vi "LinkParticles.vi"(4 "Fixed Size":bool=TRUE, 6 "Accept New":bool=TRUE, 10 "New Particle Positions":dbl[][](array[numeric])=[[305.5627746582031, 67.89103698730469], [341.9431457519531, 72.40214538574219], [232.1138153076172, 91.70089721679688], [411.30303955078125, 99.19172668457031], [201.31768798828125, 112.402099609375], [178.73162841796875, 140.29721069335938], [455.8645935058594, 155.0275421142578], [163.60015869140625, 176.1148223876953], [154.8563995361328, 211.54965209960938], [476.7146911621094, 222.72250366210938], [37.367530822753906, 236.38706970214844], [157.02395629882812, 249.5926971435547], [167.57664489746094, 281.2937927246094], [460.26348876953125, 297.98388671875], [184.57943725585938, 313.2145690917969], [442.5791320800781, 331.2660827636719], [206.3518829345703, 345.27783203125], [415.7437438964844, 355.53765869140625], [239.37156677246094, 369.4365539550781], [382.6512451171875, 372.81396484375], [268.6066589355469, 375.957275390625], [345.42205810546875, 383.692626953125], [307.2210388183594, 390.125], [315.5556335449219, 454.518798828125], [261.72613525390625, 461.53814697265625], [399.8280944824219, 466.7994079589844], [450.890869140625, 478.2618103027344]], 11 "Old Particle Positions":dbl[][](array[numeric])=[[305.5627746582031, 67.89103698730469], [341.9431457519531, 72.40214538574219], [232.1138153076172, 91.70089721679688], [411.30303955078125, 99.19172668457031], [201.31768798828125, 112.402099609375], [178.73162841796875, 140.29721069335938], [455.8645935058594, 155.0275421142578], [163.60015869140625, 176.1148223876953], [154.8563995361328, 211.54965209960938], [476.7146911621094, 222.72250366210938], [37.367530822753906, 236.38706970214844], [157.02395629882812, 249.5926971435547], [167.57664489746094, 281.2937927246094], [460.26348876953125, 297.98388671875], [184.57943725585938, 313.2145690917969], [442.5791320800781, 331.2660827636719], [206.3518829345703, 345.27783203125], [415.7437438964844, 355.53765869140625], [239.37156677246094, 369.4365539550781], [382.6512451171875, 372.81396484375], [268.6066589355469, 375.957275390625], [345.42205810546875, 383.692626953125], [307.2210388183594, 390.125], [315.5556335449219, 454.518798828125], [261.72613525390625, 461.53814697265625], [399.8280944824219, 466.7994079589844], [450.890869140625, 478.2618103027344]]) -> (3 "New Particle Positions Out":dbl[][](array[numeric]))   [LabVIEW 2017, in "ImageAcquisitionLibrary.lvlib"]
uses:
  ImageAcquisitionLibrary.lvlib
panel:
  out "Array":i32[](array[numeric])
  out "Distances":dbl[][](array[numeric])
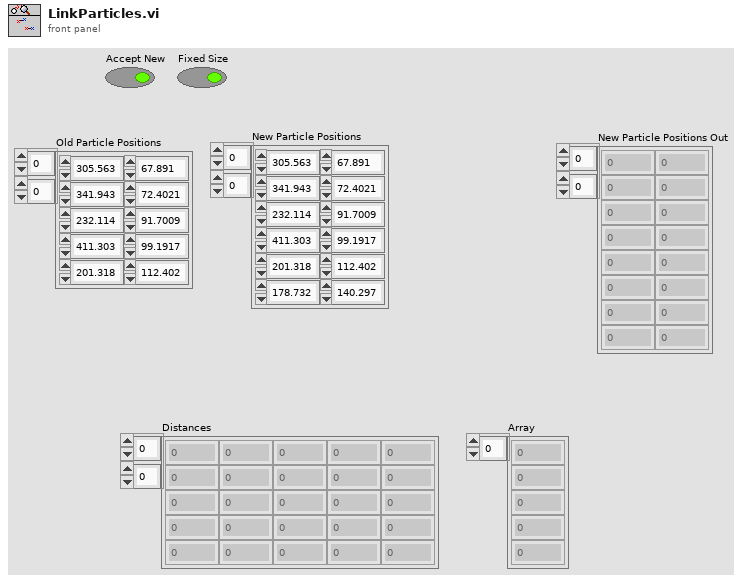
[diagram p1: front panel]
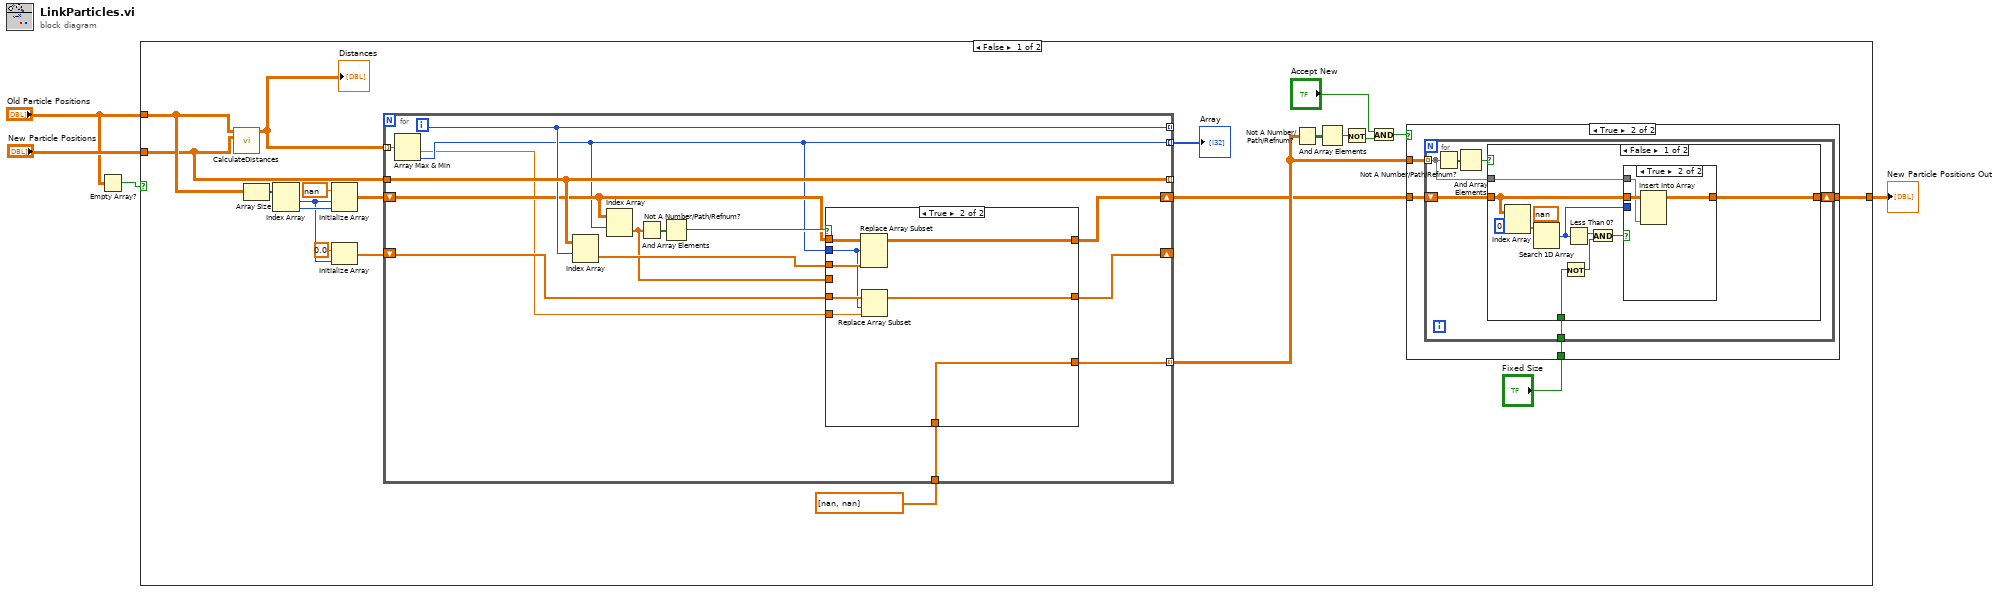
[diagram p0: block diagram]
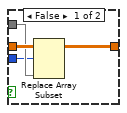
[diagram p3: hidden frame]
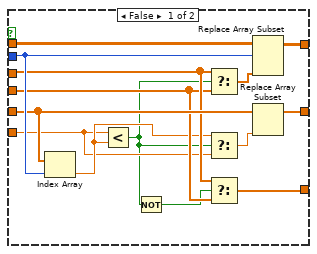
[diagram p5: hidden frame]
diagram:
  n1 = Empty Array?(array="Old Particle Positions") -> (empty?=w1:bool)
  n2 = case shown="False" w1 {
    tunnel: "Old Particle Positions" -> [w21 _]
    tunnel: "New Particle Positions" -> [w19 w93]
    tunnel: [w9 w93] -> w3
    frame False {
      n3 = call "CalculateDistances.vi"("Centroids2"=w19, "Centroids1"=w21) -> ("Distances"=w25:dbl[][])  [unwired: 9 in]
      "Distances" <- w25
      n4 = Array Size(array=w21) -> (size(s)=w23:i32[])
      n5 = Index Array(array=w23) -> (element #1=w17:i32, element #2=w24:i32)  [unwired: 2 in]
      n6 = Initialize Array(nan ("element"), w17, w24) -> (w20:dbl[][])
      n7 = Initialize Array(0.0 ("element"), w17) -> (w15:dbl[])
      n8 = for {
        tunnel: w25 -> [w70] mode=indexing
        tunnel: [w62] -> w18 mode=indexing
        tunnel: [w66] -> _ mode=indexing
        shift-right: [w63] -> w10
        shift-left: w20 -> [w64]
        tunnel: w19 -> [w67]
        tunnel: [w67] -> _ mode=indexing
        shift-right: [w59] -> _
        shift-left: w15 -> [w60]
        tunnel: [w57] -> w11 mode=indexing
        tunnel: dbl[] [nan, nan] ("New Particle Positions") -> [w56]
        i -> [w66]
        n9 = Array Max & Min(array=w70) -> (min value=w58:dbl, min index (indices)=w62:i32)  [unwired: 2 out]
        n10 = Index Array(array=w67, index (row)=w66) -> (element=w65:dbl[])  [unwired: 1 in]
        n11 = Index Array(array=w64, index (row)=w62) -> (element=w61:dbl[])  [unwired: 1 in]
        n12 = Not A Number/Path/Refnum?(number/path/refnum=w61) -> (NaN/Path/Refnum?=w69:bool[])
        n13 = And Array Elements(Boolean array=w69) -> (logical AND=w68:bool)
        n14 = case shown="True" w68 {
          tunnel: w64 -> [w84 w92]
          tunnel: w62 -> [w81 w87]
          tunnel: w65 -> [w77 w91]
          tunnel: [w83 w90] -> w63
          tunnel: w60 -> [w80 w89]
          tunnel: w61 -> [w76 _]
          tunnel: [w79 w88] -> w59
          tunnel: w58 -> [w74 w86]
          tunnel: [w71 w85] -> w57
          tunnel: w56 -> [_ w85]
          frame False {
            n15 = Index Array(array=w80, index=w81) -> (element=w75:dbl)
            n16 = Less?(x=w74, y=w75) -> (x < y?=w73:bool)
            n17 = Not(x=w73) -> (.not. x?=w72:bool)
            n18 = Select(t=w77, s=w73, f=w76) -> (s? t:f=w82:dbl[])
            n19 = Select(t=w75, s=w73, f=w74) -> (s? t:f=w78:dbl)
            n20 = Select(t=w77, s=w72, f=w76) -> (s? t:f=w71:dbl[])
            n21 = Replace Array Subset(array=w84, new element=w82, index (row)=w81) -> (w83:dbl[][])  [unwired: 1 in]
            n22 = Replace Array Subset(array=w80, new element=w78) -> (w79:dbl[])  [unwired: 1 in]
          }
          frame True {
            n23 = Replace Array Subset(array=w92, new element=w91, index (row)=w87) -> (w90:dbl[][])  [unwired: 1 in]
            n24 = Replace Array Subset(array=w89, new element=w86, index=w87) -> (w88:dbl[])
          }
        }
      }
      "Array" <- w18
      n25 = Not A Number/Path/Refnum?(number/path/refnum=w11) -> (NaN/Path/Refnum?=w13:bool[][])
      n26 = And Array Elements(Boolean array=w13) -> (logical AND=w12:bool)
      n27 = Not(x=w12) -> (.not. x?=w7:bool)
      n28 = And(x="Accept New", y=w7) -> (x .and. y?=w8:bool)
      n29 = case shown="True" w8 {
        tunnel: w11 -> [_ w30]
        tunnel: w10 -> [w26 w29]
        tunnel: [w26 w28] -> w9
        tunnel: "Fixed Size" -> [_ w27]
        frame False {
        }
        frame True {
          n30 = for {
            tunnel: w30 -> [w34] mode=indexing
            shift-right: [w32] -> w28
            shift-left: w29 -> [w33]
            tunnel: w27 -> [w31]
            n31 = Not A Number/Path/Refnum?(number/path/refnum=w34) -> (NaN/Path/Refnum?=w36:bool[])
            n32 = And Array Elements(Boolean array=w36) -> (logical AND=w35:bool)
            n33 = case shown="False" w35 {
              tunnel: w34 -> [w43 _]
              tunnel: w33 -> [w45 w55]
              tunnel: [w44 w55] -> w32
              tunnel: w31 -> [w38 _]
              frame False {
                n34 = Index Array(array=w45, index (col)=0 ("disabled index (col)")) -> (element=w47:dbl[])  [unwired: 1 in]
                n35 = Search 1D Array(1D array=w47, element=nan) -> (index of element=w41:i32)  [unwired: 1 in]
                n36 = Not(x=w38) -> (.not. x?=w37:bool)
                n37 = Less Than 0?(x=w41) -> (x < 0?=w40:bool)
                n38 = And(x=w40, y=w37) -> (x .and. y?=w39:bool)
                n39 = case shown="True" w39 {
                  tunnel: w45 -> [w51 w54]
                  tunnel: [w50 w52] -> w44
                  tunnel: w43 -> [w49 w53]
                  tunnel: w41 -> [w48 _]
                  frame False {
                    n40 = Replace Array Subset(array=w51, new element=w49, index (row)=w48) -> (w50:dbl[][])  [unwired: 1 in]
                  }
                  frame True {
                    n41 = Insert Into Array(array=w54, new element=w53) -> (w52:dbl[][])  [unwired: 2 in]
                  }
                }
              }
              frame True {
              }
            }
          }
        }
      }
    }
    frame True {
    }
  }
  "New Particle Positions Out" <- w3
